vi "Engine-Throttle-TB1.vi"(8 "Error In":errorcluster, 11 "DSI Reference":refnum<class "DCM-DSI.lvclass">) -> (0 "Error Out":errorcluster, 3 "DSI Reference":refnum<class "DCM-DSI.lvclass">)   [LabVIEW 2016, in "DSI-RT.lvlib"]
uses:
  DSI-RT.lvlib
  Classes/DCM-DSI/DCM-DSI.lvclass
  <vilib>/Powertrain Controls/Device Drivers/DCM/HH/RT/Setup.ctl
  <vilib>/Powertrain Controls/Device Drivers/DCM/HH/FPGA/Mode.ctl
  <vilib>/Powertrain Controls/Device Drivers/DCM/Rev0/FPGA/Digital Channel.ctl
  <vilib>/Powertrain Controls/Device Drivers/DCM/HH/RT/Angle Control.ctl
  <vilib>/Powertrain Controls/Device Drivers/DCM/Rev0/RT/DCM - RT.lvclass/DCM - RT.ctl
  <vilib>/Powertrain Controls/Device Drivers/DCM/HH/RT/Mode.ctl
  <vilib>/Powertrain Controls/Device Drivers/DCM/Rev0/RT/Read HH Mode.vi
  Classes/DCM-DSI/Read dt.vi
  Classes/DCM-DSI/Read HH Status.vi
  Classes/DCM-DSI/Read System ADC.vi
  Classes/DCM-DSI/Read Channels.vi
  <vilib>/Powertrain Controls/Device Drivers/Tools/Real-Time/ticks2time.vi
  Classes/DCM-DSI/Write HH Command.vi
  Classes/DCM-DSI/Write HH Chans Used.vi
  Classes/DCM-DSI/Read DCM Ref.vi
  <vilib>/addons/Software Calibration Management/xSCM/CalPoint.xnode
  <vilib>/Powertrain Controls/Device Drivers/DCM/Rev0/RT/DCM - RT.lvclass
  <vilib>/Powertrain Controls/Device Drivers/DCM/HH/RT/DCM - RT - HH.lvlib
  <vilib>/Powertrain Controls/Device Drivers/DCM/Rev0/FPGA/DCM - FPGA.lvlib
  <vilib>/Powertrain Controls/Device Drivers/DCM/HH/FPGA/DCM - FPGA - HH.lvlib
  <vilib>/addons/Software Calibration Management/xSCM/ni_scm.dll
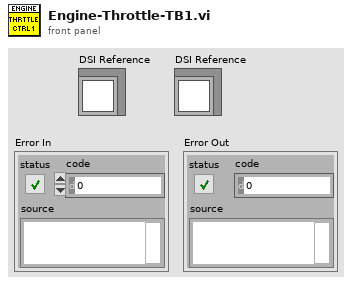
[diagram p1: front panel]
types:
  T1 = typedef "DCM - FPGA - HH.lvlib/Mode.ctl" = enum8{"Off", "Direct", "Pulse Width Modulation", "Engine Position Tracking"}
  T2 = cluster{"ModulePresent":bool, "H1Sense (A)":sgl, "H2Sense (A)":sgl, "Analog1 (V)":sgl, "Analog2 (V)":sgl, "Battery (V)":sgl, "Temperature (C)":sgl, "H1Fault":bool, "H2Fault":bool}
  T3 = typedef "DCM - RT - HH.lvlib/Setup.ctl" = cluster{"Mode":T1, "Digital Input":T4, "Polarity":bool, "Frequency [Hz]":sgl, "Duty Cycle [%]":sgl, "TDC Offset [CAD]":sgl, "Window Start [DBTDC]":sgl, "Window End [DBTDC]":sgl, "Angles":T5[], "Skip Fire":bool, "Skip Fire Index":u8}
  T4 = typedef "DCM - FPGA.lvlib/Digital Channel.ctl" = enum8{"Unused", "User OS", "Diff IO 1", "Diff IO 2", "Diff IO 3", "Diff IO 4", "Diff IO 5", "Diff IO 6", "Diff IO 7", "Diff IO 8", "Aux 1", "Aux 2", "Aux 3", "Aux 4", "Aux 5", "Aux 6", "Aux 7", "Aux 8", "Aux 9", "Aux 10", "Aux 11", "Aux 12", "Aux 13", "Aux 14", "Aux 15", "Aux 16"}
  T5 = typedef "DCM - RT - HH.lvlib/Angle Control.ctl" = cluster{"Enable":bool, "Location [DBTDC]":sgl, "Duration [s]":sgl}
  T6 = typedef "DCM - RT - HH.lvlib/Status.ctl" = cluster{"Current [A]":sgl, "Config Error":bool, "Short Fault":bool, "Open Fault":bool, "Period Min [A]":sgl, "Period Max [A]":sgl, "Period Avg [A]":sgl, "On Avg [A]":sgl}
  T7 = typedef "DCM - RT.lvclass/System ADC.ctl" = cluster{"AI 1 [V]":sgl, "AI 2 [V]":sgl, "AI 3 [V]":sgl, "AI 4 [V]":sgl, "AI 5 [V]":sgl, "AI 6 [V]":sgl, "AI 7 [V]":sgl, "AI 8 [V]":sgl, "AI 9 [V]":sgl, "AI 10 [V]":sgl, "AI 11 [V]":sgl, "AI 12 [V]":sgl, "Temp HH 1-6 [C]":sgl, "Temp HH 7-12 [C]":sgl, "Temp DI A [C]":sgl, "Temp DI Zener A [C]":sgl, "Temp DI B [C]":sgl, "Temp DI Zener B [C]":sgl, "Temp CPU [C]":sgl, "Temp Fan Intake [C]":sgl, "Temp Secondary A [C]":sgl, "Temp Primary A [C]":sgl, "Temp Boost B [C]":sgl, "Primary Range [V]":sgl, "Primary A1A2 [V]":sgl, "Primary A3A4 [V]":sgl, "Primary B3B4 [V]":sgl, "Primary B1B2 [V]":sgl, "Secondary A1A2 [V]":sgl, "Secondary A3A4 [V]":sgl, "Secondary B3B4 [V]":sgl, "Secondary B1B2 [V]":sgl, "Ext HV A [V]":sgl, "Ext HV B [V]":sgl, "FET Driver [V]":sgl, "Fan [V]":sgl, "Battery [V]":sgl, "DRVP [V]":sgl, "Key [V]":sgl, "DI Zener A [V]":sgl, "DI Zener B [V]":sgl, "Pump Zener A [V]":sgl, "Pump Zener B [V]":sgl, "MPRD [V]":sgl}
  T8 = typedef "DCM-DSI.lvclass/Channel.ctl" = cluster{"Name":string, "Unit":string, "Value":sgl}
  T9 = cluster{"Analog1 Range [V]":sgl[], "Analog2 Range [V]":sgl[], "Position Range":sgl[]}
  T10 = cluster{"TLead [sec]":sgl, "TLag [sec]":sgl, "KRpos [V/ ]":sgl, "TIpos [sec]":sgl, "TDpos [sec]":sgl, "KRneg [V/ ]":sgl, "TIneg [sec]":sgl, "TDneg [sec]":sgl, "LH Position Band":sgl, "U LH (V)":sgl, "U LH Lag [sec]":sgl, "US (V)":sgl, "US Lag [sec]":sgl, "LH Position":sgl, "Motor Resistance [Ohms]":sgl, "Position Fault Thresh":sgl}
  T11 = cluster{"Pos Cal Init Delay (sec)":sgl, "Pos Cal Return From Positive Delay (sec)":sgl, "Pos Cal Return From Negative Delay (sec)":sgl, "u Pos Cal Positive Init (V)":sgl, "u Pos Cal Negative Init (V)":sgl, "u Pos Cal Inc (V)":sgl, "u Pos Cal Dec (V)":sgl, "u Pos Cal Inc Thresh (V)":sgl, "u Pos Cal Dec Thresh (V)":sgl, "Pos Cal Offset (V)":sgl, "Pos Cal Diff Thresh (V)":sgl}
  T12 = enum16{"IDLE", "POSITION CALIBRATION", "CONTROL CALIBRATION", "CONTROL"}
  T13 = cluster{"Primary Analog Range (V)":sgl[], "Secondary Analog Range (V)":sgl[], "Position Range":sgl[], "Position Calibrated":bool, "u Pos Cal Positive (V)":sgl, "u Pos Cal Negative (V)":sgl, "u Limit Positive":bool, "u Limit Negative":bool, "Pos Cal Diff Fault":bool}
  T14 = typedef "Mode Status.ctl" = enum16{"IDLE", "POSITION CALIBRATION", "CONTROL CALIBRATION", "CONTROL"}
  T15 = cluster{"Primary Position":sgl, "Secondary Position":sgl, "AboveLH?":bool, "Position Fault":bool, "u Limit?":bool, "uLHc (V)":sgl, "uFc (V)":sgl, "uPID (V)":sgl, "u (V)":sgl}
  T16 = typedef "DCM - RT - HH.lvlib/Mode.ctl" = enum16{"Off", "Lowside", "Highside", "PFI", "Full H", "3-Phase"}
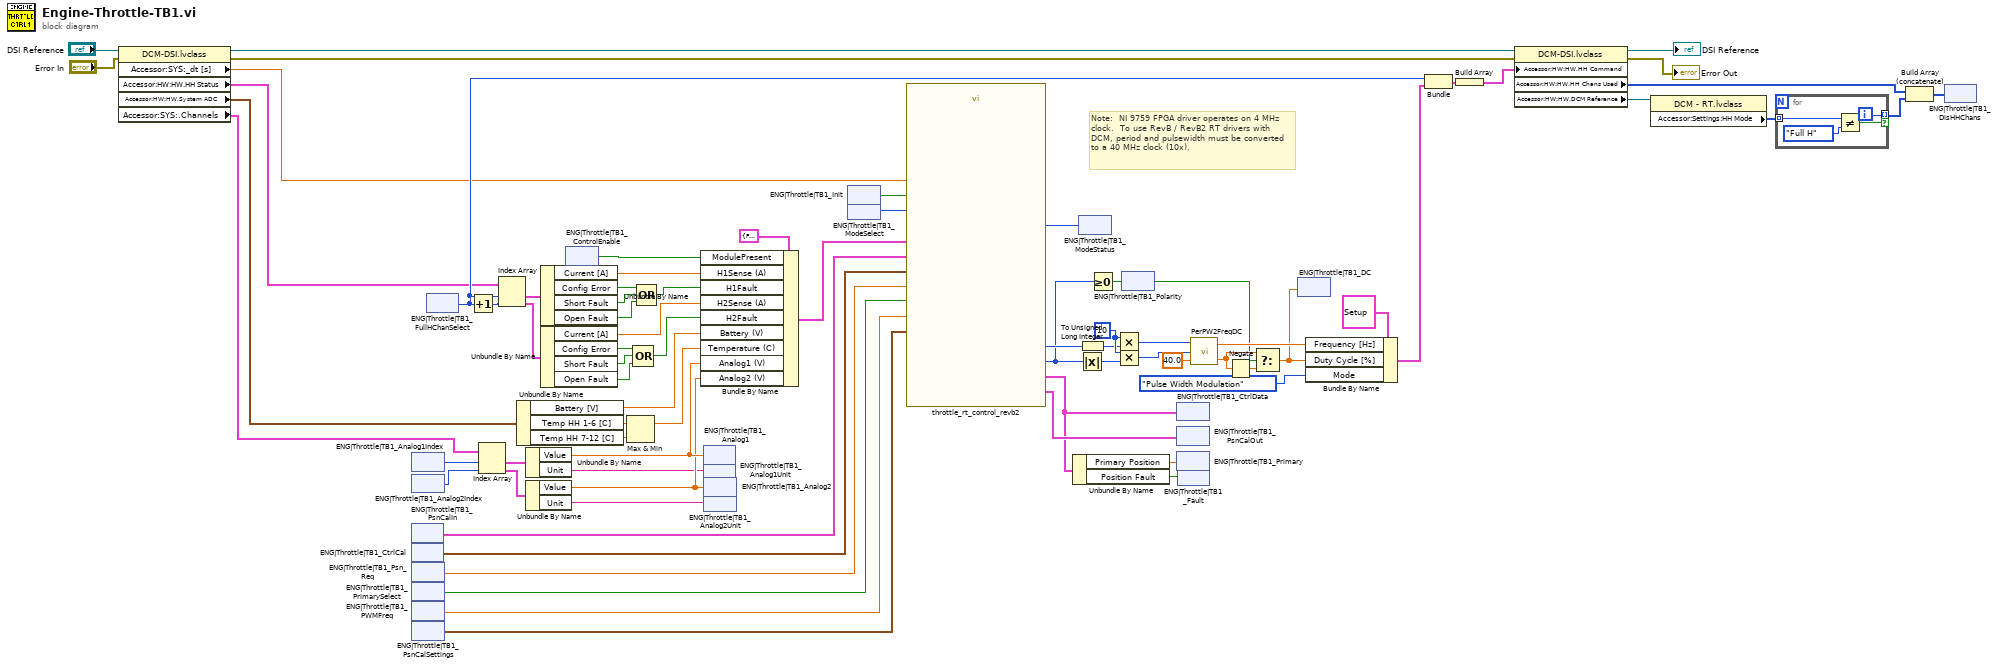
[diagram p0: block diagram]
diagram:
  w47 = u32 10 ("x")
  # "Note:  NI 9759 FPGA driver operates on 4 MHz clock.  To use RevB / RevB2 RT drivers with DCM, period and pulsewidth must be converted to a 40 MHz clock (10x)."
  n1 = property class="DCM-DSI.lvclass"(reference="DSI Reference", error in="Error In") -> (reference out=w25:refnum<class "DCM-DSI.lvclass">, error out=w24:errorcluster, "Accessor:SYS:_dt [s]"=w17:sgl, "Accessor:HW:HW.HH Status"=w14:T6[], "Accessor:HW:HW.System ADC"=w15:T7, "Accessor:SYS:.Channels"=w16:T8[])
  n2 = xnode "ENG|Throttle|TB1_PsnCalIn"() -> ("Value"=w12:T9)
  n3 = xnode "ENG|Throttle|TB1_CtrlCal"() -> ("Value"=w13:T10)
  n4 = xnode "ENG|Throttle|TB1_Analog1Index"() -> ("Value"=w75:i32)
  n5 = xnode "ENG|Throttle|TB1_Analog2Index"() -> ("Value"=w56:i32)
  n6 = xnode "ENG|Throttle|TB1_Psn_Req"() -> ("Value"=w50:sgl)
  n7 = xnode "ENG|Throttle|TB1_PrimarySelect"() -> ("Value"=w45:bool)
  n8 = xnode "ENG|Throttle|TB1_PWMFreq"() -> ("Value"=w44:sgl)
  n9 = xnode "ENG|Throttle|TB1_PsnCalSettings"() -> ("Value"=w11:T11)
  n10 = xnode "ENG|Throttle|TB1_FullHChanSelect"() -> ("Value"=w29:i32)
  n11 = Increment(x=w29) -> (x+1=w43:i32)
  n12 = Index Array(array=w16, index #1=w75, index #2=w56) -> (element #1=w42:T8, element #2=w32:T8)
  n13 = Index Array(array=w14, index #1=w29, index #2=w43) -> (element #1=w68:T6, element #2=w67:T6)
  n14 = Unbundle By Name(w15) -> ("Battery [V]"=w54:sgl, "Temp HH 1-6 [C]"=w74:sgl, "Temp HH 7-12 [C]"=w73:sgl)
  n15 = Unbundle By Name(w42) -> ("Value"=w33:sgl, "Unit"=w7:string)
  n16 = Unbundle By Name(w32) -> ("Value"=w31:sgl, "Unit"=w6:string)
  n17 = Unbundle By Name(w68) -> ("Current [A]"=w66:sgl, "Config Error"=w64:bool, "Short Fault"=w63:bool, "Open Fault"=w62:bool)
  n18 = Unbundle By Name(w67) -> ("Current [A]"=w65:sgl, "Config Error"=w60:bool, "Short Fault"=w59:bool, "Open Fault"=w58:bool)
  n19 = xnode "ENG|Throttle|TB1_ControlEnable"() -> ("Value"=w40:bool)
  n20 = Max & Min(x=w74, y=w73) -> (max(x,y)=w55:sgl)  [unwired: 1 out]
  n21 = Compound Arithmetic op=OR(w60, w59, w58) -> (w57:bool)
  n22 = Compound Arithmetic op=OR(w64, w63, w62) -> (w61:bool)
  n23 = Bundle By Name(cluster=T2 {"ModulePresent"=FALSE, "H1Sense (A)"=0.0, "H2Sense (A)"=0.0, "Analog1 (V)"=0.0, "Analog2 (V)"=0.0, "Battery (V)"=0.0, "Temperature (C)"=0.0, "H1Fault"=FALSE, "H2Fault"=FALSE} ("ThrottleDataToControl"), "ModulePresent"=w40, "H1Sense (A)"=w66, "H1Fault"=w61, "H2Sense (A)"=w65, "H2Fault"=w57, "Battery (V)"=w54, "Temperature (C)"=w55, "Analog1 (V)"=w33, "Analog2 (V)"=w31) -> (w69:T2)
  n24 = xnode "ENG|Throttle|TB1_Analog1"("Value"=w33) -> ()
  n25 = xnode "ENG|Throttle|TB1_Analog1Unit"("Value"=w7) -> ()
  n26 = xnode "ENG|Throttle|TB1_Analog2"("Value"=w31) -> ()
  n27 = xnode "ENG|Throttle|TB1_Analog2Unit"("Value"=w6) -> ()
  n28 = xnode "ENG|Throttle|TB1_Init"() -> ("Value"=w39:bool)
  n29 = xnode "ENG|Throttle|TB1_ModeSelect"() -> ("Value"=w8:T12)
  n30 = call <vilib>:"throttle_rt_control_revb2.vi"("Mode Request"=w8, "Module Data"=w69, "Primary Position (F=1, T=2)"=w45, "PWM Frequency (Hz)"=w44, "Position Setpoint"=w50, "dt (sec)"=w17, "Position Cal Settings"=w11, "Position Cal In"=w12, "Control Cal In"=w13, "initialize"=w39) -> ("Position Cal Out"=w10:T13, "Mode Status"=w9:T14, "Control Data"=w5:T15, "Throttle Period Ticks"=w51:u16, "Throttle Pulse Width Ticks"=w49:i16)  [unwired: 4 in, 1 out]
  n31 = Unbundle By Name(w5) -> ("Primary Position"=w4:sgl, "Position Fault"=w3:bool)
  n32 = xnode "ENG|Throttle|TB1_ModeStatus"("Value"=w9) -> ()
  n33 = To Unsigned Long Integer(number=w51) -> (unsigned 32bit integer=w46:u32)
  n34 = Absolute Value(x=w49) -> (abs(x)=w48:i16)
  n35 = Greater Or Equal To 0?(x=w49) -> (x >= 0?=w35:bool)
  n36 = Multiply(x=w47, y=w46) -> (x*y=w53:u32)
  n37 = Multiply(x=w47, y=w48) -> (x*y=w52:u32)
  n38 = xnode "ENG|Throttle|TB1_Polarity"("Value"=w35) -> ()
  n39 = xnode "ENG|Throttle|TB1_CtrlData"("Value"=w5) -> ()
  n40 = xnode "ENG|Throttle|TB1_PsnCalOut"("Value"=w10) -> ()
  n41 = xnode "ENG|Throttle|TB1_Primary"("Value"=w4) -> ()
  n42 = xnode "ENG|Throttle|TB1_Fault"("Value"=w3) -> ()
  n43 = call <vilib>:"PerPW2FreqDC.vi"("Clock Frequency (MHz, 40)"=sgl 40.0, "PulseWidth(ticks)"=w52, "Period(ticks)"=w53) -> ("DutyCycle(%)"=w36:sgl, "Frequency(Hz)"=w41:sgl)
  n44 = Negate(x=w36) -> (-x=w37:sgl)
  n45 = Select(t=w36, s=w35, f=w37) -> (s? t:f=w38:sgl)
  n46 = xnode "ENG|Throttle|TB1_DC"("Value"=w38) -> ()
  n47 = Bundle By Name(cluster=T3 {"Mode"=enum."Off", "Digital Input"=enum."Unused", "Polarity"=FALSE, "Frequency [Hz]"=0.0, "Duty Cycle [%]"=0.0, "TDC Offset [CAD]"=0.0, "Window Start [DBTDC]"=0.0, "Window End [DBTDC]"=0.0, "Angles"=[{"Enable"=FALSE, "Location [DBTDC]"=0.0, "Duration [s]"=0.0}, {"Enable"=FALSE, "Location [DBTDC]"=0.0, "Duration [s]"=0.0}, {"Enable"=FALSE, "Location [DBTDC]"=0.0, "Duration [s]"=0.0}, {"Enable"=FALSE, "Location [DBTDC]"=0.0, "Duration [s]"=0.0}], "Skip Fire"=FALSE, "Skip Fire Index"=0} ("element"), "Frequency [Hz]"=w41, "Duty Cycle [%]"=w38, "Mode"=Mode."Pulse Width Modulation") -> (w28:T3)
  n48 = Bundle("Value"=w29, "element"=w28) -> (w27:cluster{"Value":i32, "element":T3})  [unwired: 1 in]
  n49 = Build Array(w27) -> (w19:cluster{"Value":i32, "element":T3}[])
  n50 = property class="DCM-DSI.lvclass"(reference=w25, error in=w24, "Accessor:HW:HW.HH Command"=w19) -> (reference out=→"DSI Reference":refnum<class "DCM-DSI.lvclass">, error out=→"Error Out":errorcluster, "Accessor:HW:HW.HH Chans Used"=w1:i32[], "Accessor:HW:HW.DCM Reference"=w2:refnum<class "DCM - RT.lvclass">)
  n51 = property class="DCM - RT.lvclass"(reference=w2) -> ("Accessor:Settings:HH Mode"=w26:T16[])  [unwired: 1 in, 2 out]
  n52 = for {
    tunnel: [w78] -> w18 mode=indexing if=w77
    tunnel: w26 -> [w76] mode=indexing
    i -> [w78]
    n53 = Not Equal?(x=w76, y=Mode."Full H" ("Mode")) -> (x != y?=w77:bool)
  }
  n54 = Build Array (concatenate)(w1, w18) -> (w71:i32[])
  n55 = xnode "ENG|Throttle|TB1_DisHHChans"("Value"=w71) -> ()
